vi "Set Current.vi"(5 "Vout5_Res":dbl=100000.0 format="%#_13g", 6 "SWIR?":bool, 7 "Vout3_Res":dbl=10000000.0 format="%#_13g", 8 "error in (no error)":errorcluster, 9 "Current":dbl, 10 "task in":refnum<k24>) -> (0 "error out":errorcluster, 2 "task out":refnum<k24>)   [LabVIEW 2025]
uses:
  <instrlib>/ULx/ULx_LV.dll
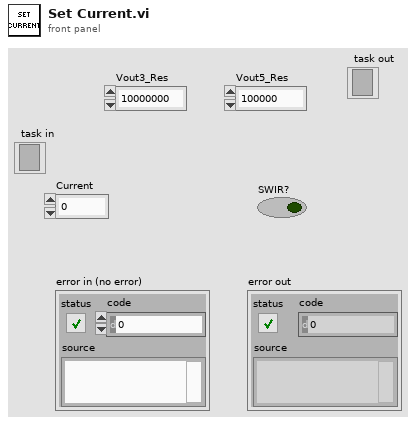
[diagram p1: front panel]
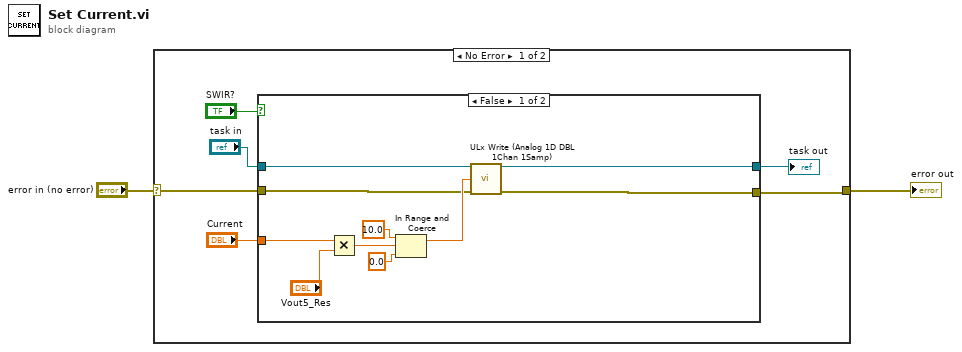
[diagram p0: block diagram]
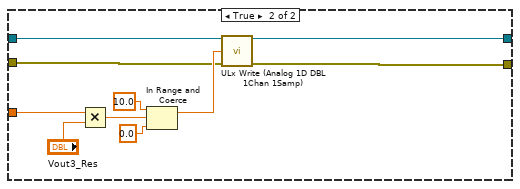
[diagram p2: hidden frame]
diagram:
  n1 = case shown="No Error" "error in (no error)" {
    selector: "error in (no error)" -> [w8 w29]
    tunnel: [w7 w29] -> w1
    frame No Error {
      n2 = case shown="False" "SWIR?" {
        tunnel: w8 -> [w12 w22]
        tunnel: [w11 w21] -> w7
        tunnel: "Current" -> [w18 w28]
        tunnel: "task in" -> [w10 w20]
        tunnel: [w9 w19] -> w3
        frame False {
          n3 = Multiply(x=w18, y="Vout5_Res") -> (x*y=w16:dbl)
          n4 = In Range and Coerce(upper limit=10.0, x=w16, lower limit=0.0) -> (coerced(x)=w13:dbl)  [unwired: 1 out]
          n5 = call <instrlib>:"ULx Write (Analog 1D DBL 1Chan 1Samp).vi"("task in"=w10, "data"=w13, "error in"=w12) -> ("task out"=w9:refnum<k24>, "error out"=w11:errorcluster)  [unwired: 10 in, 1 out]
        }
        frame True {
          n6 = Multiply(x=w28, y="Vout3_Res") -> (x*y=w26:dbl)
          n7 = In Range and Coerce(upper limit=10.0, x=w26, lower limit=0.0) -> (coerced(x)=w23:dbl)  [unwired: 1 out]
          n8 = call <instrlib>:"ULx Write (Analog 1D DBL 1Chan 1Samp).vi"("task in"=w20, "data"=w23, "error in"=w22) -> ("task out"=w19:refnum<k24>, "error out"=w21:errorcluster)  [unwired: 10 in, 1 out]
        }
      }
      "task out" <- w3
    }
    frame Error {
    }
  }
  "error out" <- w1
